vi "Get Thread Parameters.vi"(11 "Transceiver Thread in":refnum<class "Transceiver Thread.lvclass">) -> (2 "Thread Parameters":refnum<class "Thread Parameters.lvclass">, 3 "Transceiver Thread out":refnum<class "Transceiver Thread.lvclass">)   [LabVIEW 2017, in "Data Sharing Framework Engine.lvlib" / "Transceiver Thread.lvclass"]
uses:
  Transceiver Thread.lvclass
  old/dsf core/Source/Engine/Classes/Thread Parameters/Thread Parameters.lvclass
  Transceiver Thread.lvclass/Transceiver Thread.ctl
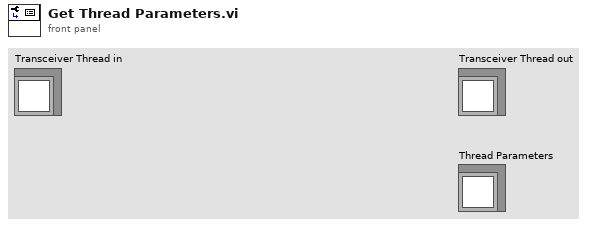
[diagram p1: front panel]
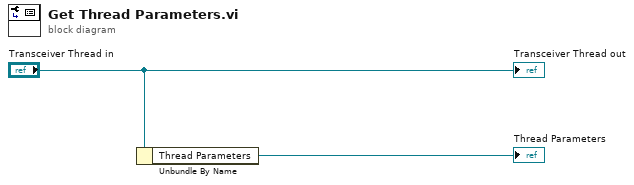
[diagram p0: block diagram]
diagram:
  n1 = Unbundle By Name("Transceiver Thread in") -> ("Thread Parameters"=→"Thread Parameters":refnum<class "Thread Parameters.lvclass">)
  "Transceiver Thread out" <- "Transceiver Thread in"
